vi "CREA PROFILI.vi"() -> ()   [LabVIEW 2019]
panel:
  in  "NOME PROFILO":string
  in  "EXIT":bool
  in  "INSERT STEP":bool
  in  "Multicolumn Listbox":i32(listbox)
  in  "STEP GENERICO":T1
  in  "TIPO PROFILO":u16(ring) items=["TERMICA", "TRASCINAMENTO", "CARICO", "VUOTO"]
  in  "NUMERO ALIMENTATORI":enum32{"TRIFASE", "MONOFASE"}(radio)
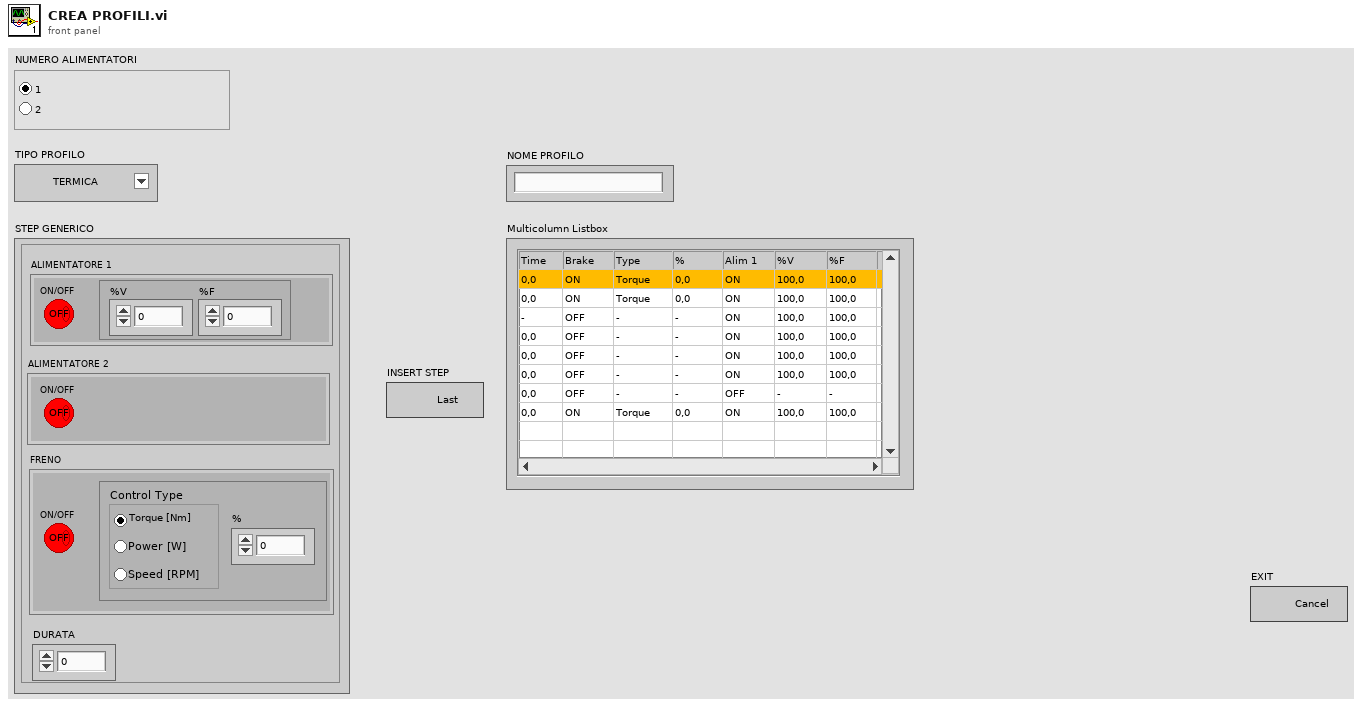
[diagram p1: front panel]
types:
  T1 = cluster{"ALIMENTATORE 1":cluster{"ON/OFF":bool, "SET":cluster{"%V":dbl, "%F":dbl}}, "FRENO":cluster{"ON/OFF":bool, "SET":cluster{"%":dbl, "Control Type":enum32{"Torque [Nm]", "Power [W]", "Speed [RPM]"}}}, "DURATA":dbl, "ALIMENTATORE 2":cluster{"ON/OFF":bool, "SET":cluster{"%V":dbl, "%F":dbl}}}
  T2 = enum32{"Torque [Nm]", "Power [W]", "Speed [RPM]"}
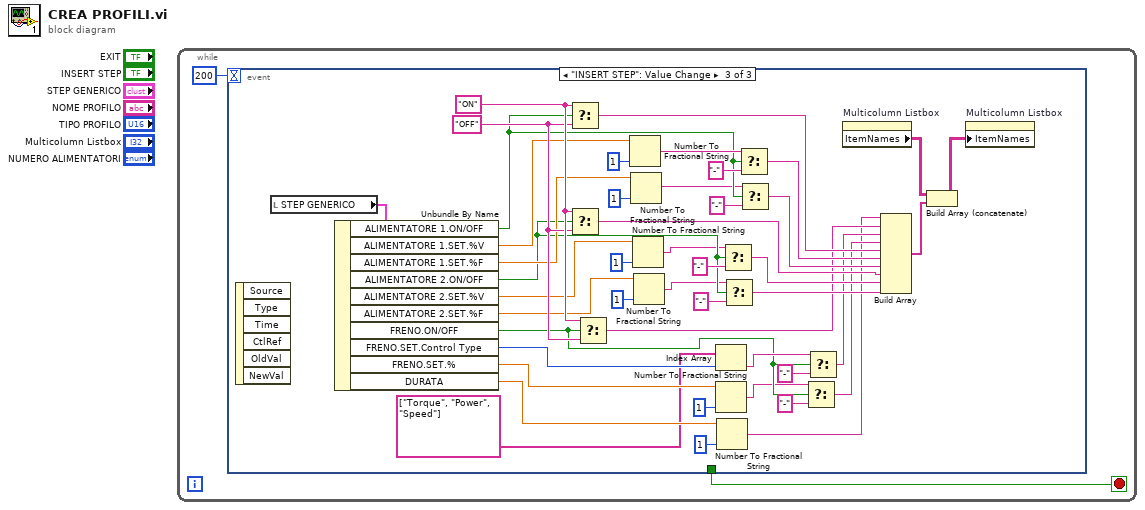
[diagram p0: block diagram]
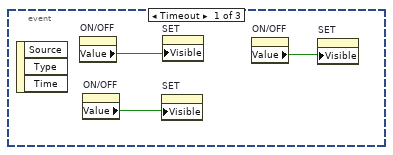
[diagram p2: hidden frame]
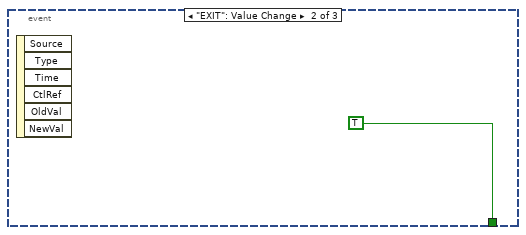
[diagram p3: hidden frame]
diagram:
  n1 = while {
    stop <- w1 stop-if-true
    n2 = event shown="[2] \"INSERT STEP\": Value Change" {
      selector: _ -> [_ _ _]
      dyn-events: _ -> [_ _ _]
      timeout: 200 -> [_ _ _]
      tunnel: [_ TRUE _] -> w1
      event Timeout {
        n3 = event-data() -> ()  [unwired: 1 in, 3 out]
        n4 = property on="ON/OFF" class="Bool (strict)"() -> ("Value"=w5:bool)  [unwired: 2 in, 2 out]
        n5 = property on="ON/OFF" class="Bool (strict)"() -> ("Value"=w4:bool)  [unwired: 2 in, 2 out]
        n6 = property on="SET" class="Clust (strict)"("Visible"=w4) -> ()  [unwired: 2 in, 2 out]
        n7 = property on="SET" class="Clust (strict)"("Visible"=w5) -> ()  [unwired: 2 in, 2 out]
        n8 = property on="ON/OFF" class="Bool (strict)"() -> ("Value"=w3:bool)  [unwired: 2 in, 2 out]
        n9 = property on="SET" class="Clust (strict)"("Visible"=w3) -> ()  [unwired: 2 in, 2 out]
      }
      event "EXIT": Value Change {
        n10 = event-data() -> ()  [unwired: 1 in, 6 out]
      }
      event "INSERT STEP": Value Change {
        w49 = "OFF" ("f")
        w50 = "ON"
        n11 = event-data() -> ()  [unwired: 1 in, 6 out]
        n12 = local read "STEP GENERICO"() -> (w51:T1)
        n13 = Unbundle By Name(w51) -> ("ALIMENTATORE 1.ON/OFF"=w23:bool, "ALIMENTATORE 1.SET.%V"=w36:dbl, "ALIMENTATORE 1.SET.%F"=w35:dbl, "ALIMENTATORE 2.ON/OFF"=w16:bool, "ALIMENTATORE 2.SET.%V"=w34:dbl, "ALIMENTATORE 2.SET.%F"=w33:dbl, "FRENO.ON/OFF"=w31:bool, "FRENO.SET.Control Type"=w40:T2, "FRENO.SET.%"=w42:dbl, "DURATA"=w41:dbl)
        n14 = Select(t=w50, s=w23, f=w49) -> (s? t:f=w27:string)
        n15 = Select(t=w50, s=w16, f=w49) -> (s? t:f=w17:string)
        n16 = Select(t=w50, s=w31, f=w49) -> (s? t:f=w8:string)
        n17 = Number To Fractional String(number=w36, precision (6)=i16 1) -> (F-format string=w25:string)  [unwired: 2 in]
        n18 = Number To Fractional String(number=w35, precision (6)=i16 1) -> (F-format string=w22:string)  [unwired: 2 in]
        n19 = Number To Fractional String(number=w34, precision (6)=i16 1) -> (F-format string=w15:string)  [unwired: 2 in]
        n20 = Number To Fractional String(number=w33, precision (6)=i16 1) -> (F-format string=w14:string)  [unwired: 2 in]
        n21 = Index Array(array=string[] ["Torque", "Power", "Speed"], index=w40) -> (element=w32:string)
        n22 = Number To Fractional String(number=w42, precision (6)=i16 1) -> (F-format string=w30:string)  [unwired: 2 in]
        n23 = Number To Fractional String(number=w41, precision (6)=i16 1) -> (F-format string=w7:string)  [unwired: 2 in]
        n24 = Select(t=w15, s=w16, f="-") -> (s? t:f=w13:string)
        n25 = Select(t=w14, s=w16, f="-") -> (s? t:f=w12:string)
        n26 = Select(t=w25, s=w23, f="-") -> (s? t:f=w21:string)
        n27 = Select(t=w22, s=w23, f="-") -> (s? t:f=w20:string)
        n28 = Select(t=w30, s=w31, f="-") -> (s? t:f=w10:string)
        n29 = Select(t=w32, s=w31, f="-") -> (s? t:f=w9:string)
        n30 = property on="Multicolumn Listbox" class="MCListbox (strict)"() -> ("ItemNames"=w38:string[][])  [unwired: 2 in, 2 out]
        n31 = Build Array(w7, w8, w9, w10, w27, w21, w20, w17, w13, w12) -> (w11:string[])
        n32 = Build Array (concatenate)(w38, w11) -> (w37:string[][])
        n33 = property on="Multicolumn Listbox" class="MCListbox (strict)"("ItemNames"=w37) -> ()  [unwired: 2 in, 2 out]
      }
    }
  }
